vi "PH_PSDBWriter.Wrap Image Data.vi"(1 "Unit Array":string[](array[string]), 2 "Data Arrray":T2[](array[typedef]), 3 "Name Array":string[](array[string]), 4 "Name Prefix":string) -> (0 "PSDB Image Data Array":T1[](array[typedef]))   [LabVIEW 2014, in "PH_PSDBWriter.lvlib"]
uses:
  PH_PSDBWriter.lvlib
  <vilib>/vision/Image Controls.llb/IMAQ Image.ctl
  PH_PSDBWriter.Image dataset.ctl
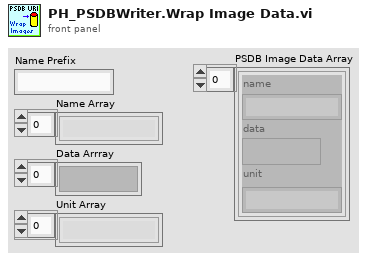
[diagram p1: front panel]
types:
  T1 = typedef "PH_PSDBWriter.lvlib/PH_PSDBWriter.Image dataset.ctl" = cluster{"name":string, "data":T2, "unit":string}
  T2 = typedef "IMAQ Image.ctl" = refnum<image>
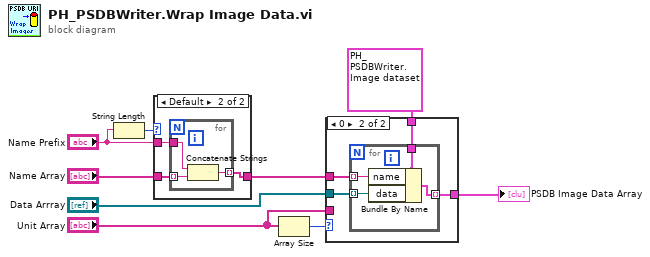
[diagram p0: block diagram]
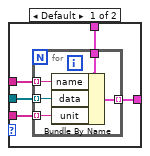
[diagram p2: hidden frame]
diagram:
  n1 = String Length(string="Name Prefix") -> (length=w6:i32)
  n2 = case shown="Default" w6 {
    tunnel: "Name Array" -> [w10 w13]
    tunnel: [w10 w11] -> w3
    tunnel: "Name Prefix" -> [_ w12]
    frame 0 {
    }
    frame Default {
      n3 = for {
        tunnel: w13 -> [w16] mode=indexing
        tunnel: w12 -> [w15]
        tunnel: [w14] -> w11 mode=indexing
        n4 = Concatenate Strings(w15, w16) -> (w14:string)
      }
    }
  }
  n5 = Array Size(array="Unit Array") -> (size(s)=w1:i32)
  n6 = case shown="0" w1 {
    tunnel: T1 {"name"="", "data"="untitled", "unit"=""} ("Image data") -> [w21 w30]
    tunnel: "Data Arrray" -> [w20 w29]
    tunnel: [w19 w28] -> w7
    tunnel: w3 -> [w18 w27]
    tunnel: "Unit Array" -> [w17 _]
    frame Default {
      n7 = for {
        tunnel: w21 -> [w26]
        tunnel: [w25] -> w19 mode=indexing
        tunnel: w20 -> [w24] mode=indexing
        tunnel: w18 -> [w23] mode=indexing
        tunnel: w17 -> [w22] mode=indexing
        n8 = Bundle By Name(cluster=w26, "name"=w23, "data"=w24, "unit"=w22) -> (w25:T1)
      }
    }
    frame 0 {
      n9 = for {
        tunnel: w30 -> [w34]
        tunnel: [w33] -> w28 mode=indexing
        tunnel: w29 -> [w32] mode=indexing
        tunnel: w27 -> [w31] mode=indexing
        n10 = Bundle By Name(cluster=w34, "name"=w31, "data"=w32) -> (w33:T1)
      }
    }
  }
  "PSDB Image Data Array" <- w7
